vi "SpeakerTask2ndEar.vi"(0 "stop":bool, 4 "path":path=path "E:/Code/Labview/SoundIdentity/Sounds/Test/TestANJALI.wav") -> (1 "Waveform Graph":waveform(dbl)[](graph)=[{"t0"=timestamp(0 s since 1904-01-01), "dt"=6.25e-05, "Y"=array[16640 elements]}])   [LabVIEW 2010]
doc: "I. Description:\nThis example demonstrates how to output a continuous periodic waveform using an internal sample clock.\n\nII. Instructions for Running:\n1. Select the Physical Channel to correspond to where your signal is output on the DAQ device.\n2. Enter the Minimum and Maximum Voltage Ranges\n3. Specify the Desired Frequency of the output Waveform\n4. Enter the Waveform Information. See the documentation of the Waveform Buffer Generation SubVI for information on each parameter.\n\nIII. Block Diagram Steps:\n1. Create an Analog Output Voltage channel.\n2. Call the DAQmx Timing (Use Waveform) VI which sets the sample clock rate based on the input waveform parameters, and set the sample mode to Continuous.\n3. Write the waveform to the output buffer.\n4. Call the Start VI.\n5. Loop continuously until the user presses the Stop button. Check for errors every 100 ms using the Is Task Done? VI\n6. Clear the Task\n7. Use the popup dialog box to display an error or warning if any.\n\nIV. I/O Connections Overview:\nMake sure your signal output terminal matches the Physical Channel I/O Control. For further connection information, refer to your hardware reference manual."
uses:
  <vilib>/Utility/error.llb/DialogType.ctl
  <vilib>/DAQmx/write.llb/DAQmx Write (Analog 1D DBL 1Chan NSamp).vi
  <vilib>/DAQmx/configure/timing.llb/DAQmx Timing (Sample Clock).vi
  <vilib>/measure/maspectr.llb/FFT Power Spectrum for N Chan.vi
  <vilib>/daqmx/miscellaneous.llb/DAQmx Fill In Error Info.vi
  <vilib>/measure/NI_MAPro.lvlib
panel:
  in  "Power Spectrum":bool
  out "Power Spectrum 2":cluster{"f0":dbl, "df":dbl, "magnitude":dbl[]}[](graph)
  out "Done":bool=TRUE
  out "Completed":dbl=1.0 format="%0.0f"
  in  "restart":bool
  in  "dB":bool=TRUE
  in  "stop 2":bool
  in  "window":T1(ring)=enum."Hanning"
  in  "averaging parameters":T2={"averaging mode"=enum."No averaging", "weighting mode"=enum."Exponential", "number of averages"=10} {"number of averages" min=1}
  # "Real-Time Spectral Measurements"
  # "Sampling Rate"
  # "Wav File"
  # "Channel Parameters"
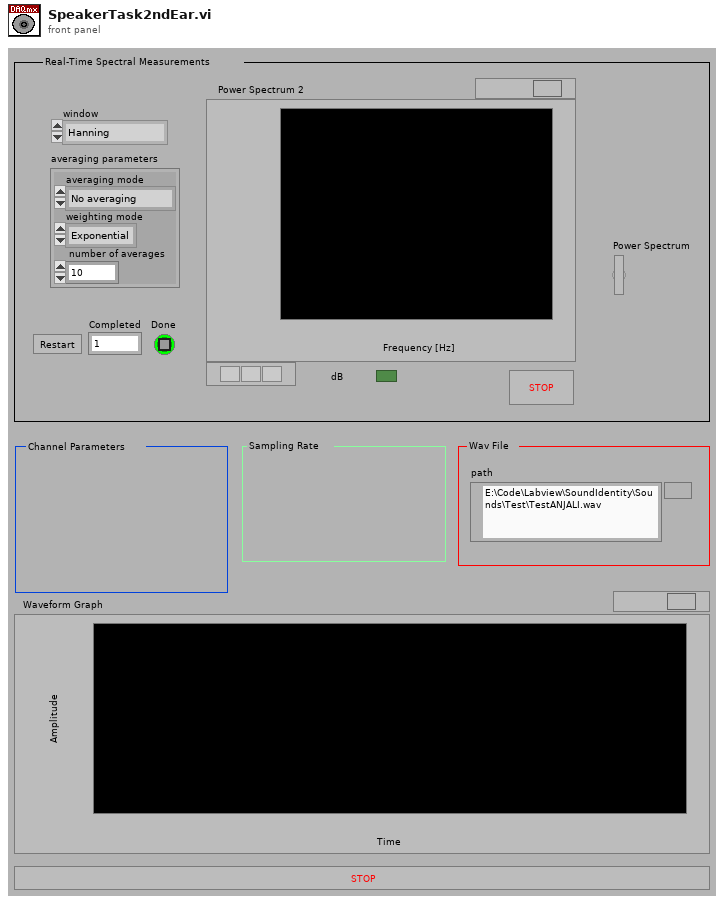
[diagram p1: front panel]
types:
  T1 = enum16{"None ", "Hanning", "Hamming", "Blackman-Harris", "Exact Blackman", "Blackman", "Flat Top", "4 Term B-Harris ", "7 Term B-Harris", "Low Sidelobe"}
  T2 = cluster{"averaging mode":enum16{"No averaging", "Vector averaging", "RMS averaging", "Peak hold"}, "weighting mode":enum16{"Linear", "Exponential"}, "number of averages":u32}
  T3 = typedef "DialogType.ctl" = u16
  T4 = cluster{"data[0]":waveform(dbl), "data[1]":waveform(dbl), "data[2]":waveform(dbl), "data[3]":waveform(dbl), "data[4]":waveform(dbl), "data[5]":waveform(dbl), "data[6]":waveform(dbl), "data[7]":waveform(dbl), "data[8]":waveform(dbl)}
  T5 = enum16{"Initialize", "String", "Start", "New Session", "Stop", "Resume", "Close"}
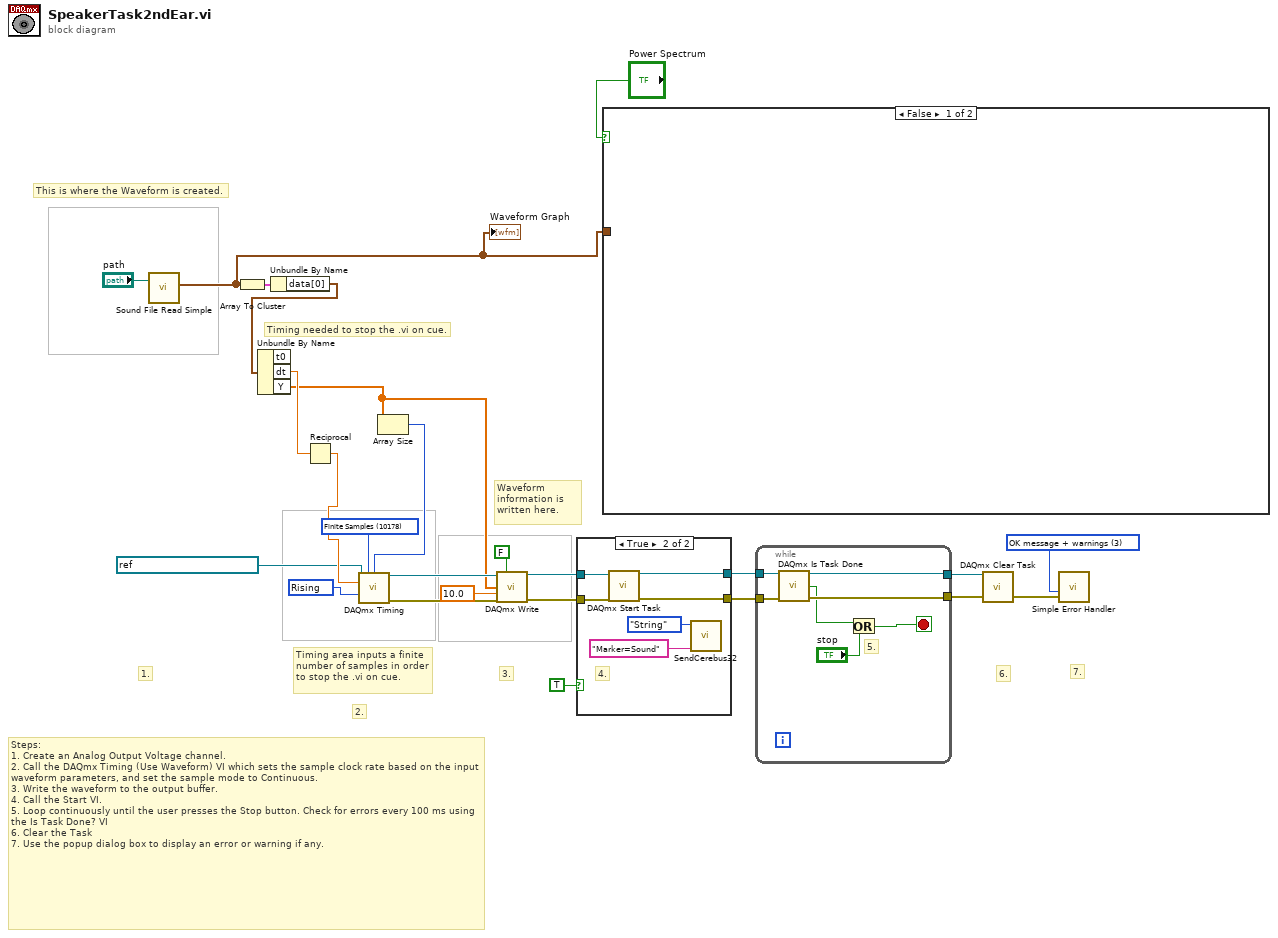
[diagram p0: block diagram]
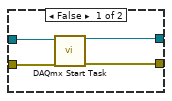
[diagram p2: hidden frame]
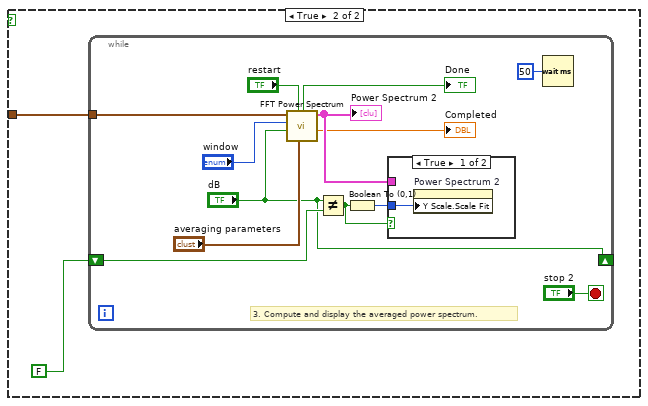
[diagram p3: hidden frame]
diagram:
  w13 = 10280 items=["Rising"=10280, "Falling"=10171] ("active edge")
  w16 = T3 3 items=["no dialog", "OK message", "continue or stop message", "OK message + warnings", "continue/stop + warnings"] ("type of dialog (OK msg:1)")
  w24 = 10178 items=["Finite Samples"=10178, "Continuous Samples"=10123] ("sample mode")
  # "Waveform information is written here."
  # "Timing area inputs a finite number of samples in order to stop the .vi on cue."
  # "Timing needed to stop the .vi on cue."
  # "This is where the Waveform is created."
  # "7."
  # "6."
  # "Steps: \n1. Create an Analog Output Voltage channel.\n2. Call the DAQmx Timing (Use Waveform) VI which sets the sample clock rate based on the input waveform parameters, and set the sample mode to Continuous.\n3. Write the waveform to the output buffer.\n4. Call the Start VI.\n5. Loop continuously until the user presses the Stop button. Check for errors every 100 ms using the Is Task Done? VI\n6. Clear the Task\n7. Use the popup dialog box to display an error or warning if any."
  # "3."
  # "2."
  # "1."
  n1 = call <vilib>:"Sound File Read Simple.vi"("path"="path") -> ("data"=w6:waveform(dbl)[])  [unwired: 7 in, 3 out]
  "Waveform Graph" <- w6
  n2 = Array To Cluster(array=w6) -> (cluster=w8:T4)
  n3 = Unbundle By Name(w8) -> ("data[0]"=w7:waveform(dbl))
  n4 = Unbundle By Name(w7) -> ("dt"=w4:dbl, "Y"=w2:dbl[])  [unwired: 1 out]
  n5 = Reciprocal(x=w4) -> (1/x=w3:dbl)
  n6 = Array Size(array=w2) -> (size(s)=w5:i32)
  n7 = call-poly <vilib>:"DAQmx Timing.vi"("task/channels in"=refnum<k21> "make_sound_other_ear", "sample mode"=w24, "samples per channel"=w5, "rate"=w3, "active edge"=w13) -> ("task out"=w19:refnum<k21>, "error out"=w18:errorcluster)  [unwired: 9 in]
  n8 = call-poly <vilib>:"DAQmx Write.vi"("task/channels in"=w19, "auto start"=FALSE, "data"=w2, "timeout"=10.0 ("Wirite Timeout"), "error in"=w18) -> ("task out"=w23:refnum<k21>, "error out"=w22:errorcluster)  [unwired: 8 in, 1 out]
  n9 = case shown="True" TRUE {
    tunnel: w23 -> [w29 w35]
    tunnel: w22 -> [w28 w34]
    tunnel: [w26 w33] -> w20
    tunnel: [w27 w32] -> w17
    frame False {
      n10 = call <vilib>:"DAQmx Start Task.vi"("task/channels in"=w29, "error in"=w28) -> ("task out"=w27:refnum<k21>, "error out"=w26:errorcluster)  [unwired: 12 in]
    }
    frame True {
      # "4."
      n11 = call <vilib>:"DAQmx Start Task.vi"("task/channels in"=w35, "error in"=w34) -> ("task out"=w32:refnum<k21>, "error out"=w33:errorcluster)  [unwired: 12 in]
      n12 = call "SendCerebus32.vi"("String"="Marker=Sound" ("ASCII Data"), "Mode"=T5."String") -> ()  [unwired: 3 in]
    }
  }
  n13 = case shown="False" "Power Spectrum" {
    tunnel: w6 -> [_ w36]
    frame False {
    }
    frame True {
      n14 = while {
        shift-left: FALSE ("dB") -> [w44]
        shift-right: ["dB"] -> _
        tunnel: w36 -> [w38]
        stop <- "stop 2" stop-if-true
        # "3. Compute and display the averaged power spectrum."
        n15 = call-poly <vilib>:"FFT Power Spectrum.vi"("averaging parameters"="averaging parameters", "restart averaging (F)"="restart", "dB On (F)"="dB", "window"="window", "time signals"=w38) -> ("averages completed"=→"Completed":dbl, "power spectra"=w48:cluster{"f0":dbl, "df":dbl, "magnitude":dbl[]}[], "averaging done"=→"Done":bool)  [unwired: 3 in, 1 out]
        "Power Spectrum 2" <- w48
        n16 = Not Equal?(x="dB", y=w44) -> (x != y?=w43:bool)
        n17 = Boolean To (0,1)(Boolean=w43) -> (0, 1=w42:i16)
        n18 = case shown="True" w43 {
          tunnel: w42 -> [w51 _]
          tunnel: w48 -> [_ _]
          frame True {
            n19 = property on="Power Spectrum 2" class="WFGraph (strict)"("Y Scale.Scale Fit"=w51) -> ()  [unwired: 2 in, 2 out]
          }
          frame False {
          }
        }
        n20 = Wait (ms)(milliseconds to wait=u32 50 ("millisecond multiple")) -> ()  [unwired: 1 out]
      }
    }
  }
  n21 = while {
    tunnel: w17 -> [w58]
    tunnel: [w57] -> w15
    tunnel: w20 -> [w56]
    tunnel: [w55] -> w14
    stop <- w54 stop-if-true
    # "5."
    n22 = call <vilib>:"DAQmx Is Task Done.vi"("task/channels in"=w58, "error in"=w56) -> ("task out"=w57:refnum<k21>, "task done?"=w52:bool, "error out"=w55:errorcluster)  [unwired: 11 in]
    n23 = Or(x=w52, y="stop") -> (x .or. y?=w54:bool)
  }
  n24 = call <vilib>:"DAQmx Clear Task.vi"("task in"=w15, "error in"=w14) -> ("error out"=w25:errorcluster)  [unwired: 13 in]
  n25 = call <vilib>:"Simple Error Handler.vi"("type of dialog (OK msg:1)"=w16, "error in (no error)"=w25) -> ()  [unwired: 3 in, 5 out]
